vi "AUTOFLIM_Fine_Alignment.vi"(0 "System no.":i32, 5 "Scan Termination":T1(ring)=enum."Center of scan", 11 "error in":errorcluster) -> (4 "Mesh out":dbl, 6 "Numeric 2":dbl, 8 "Numeric":dbl, 10 "Alignment Array Out":dbl[][](array[numeric]), 15 "error out":errorcluster)   [LabVIEW 2023]
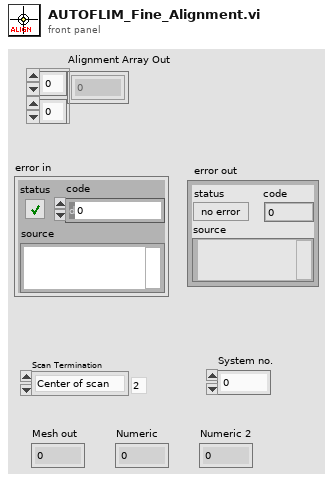
[diagram p1: front panel]
types:
  T1 = enum16{"Maximum", "End Position", "Center of scan"}
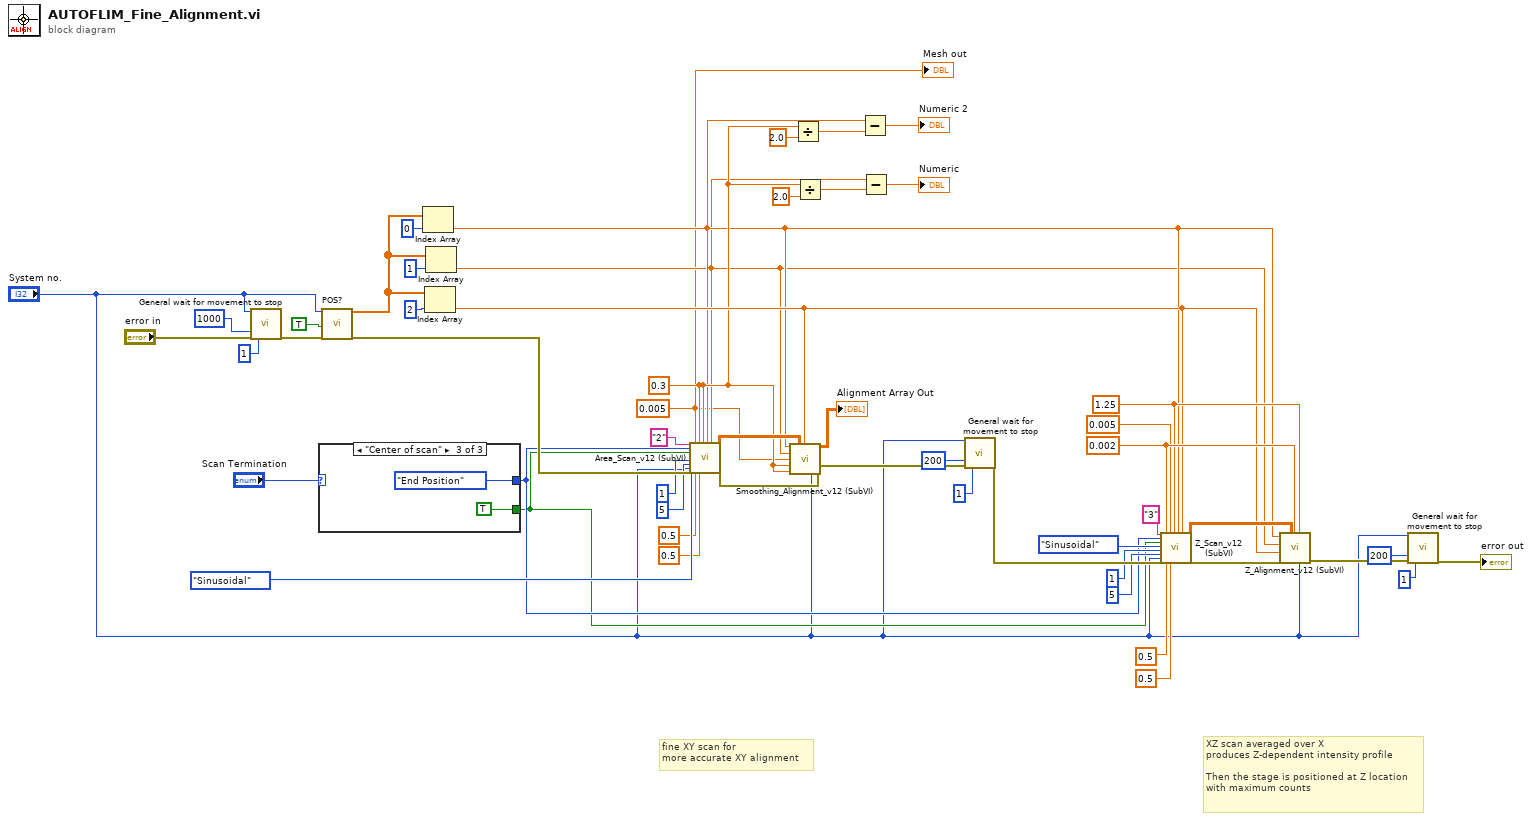
[diagram p0: block diagram]
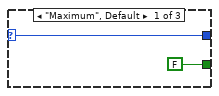
[diagram p2: hidden frame]
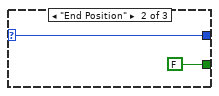
[diagram p3: hidden frame]
diagram:
  w23 = 0.002 ("Z Mesh")
  w21 = 1.25 ("Z range")
  w10 = 0.3
  w1 = 0.005
  # "fine XY scan for\nmore accurate XY alignment"
  # "XZ scan averaged over X\nproduces Z-dependent intensity profile\n\nThen the stage is positioned at Z location\nwith maximum counts"
  n1 = call "General wait for movement to stop.vi"("System no."="System no.", "Additional wait time, ms"=1000, "error in"="error in", "Polling cycle \ntime, ms"=1) -> ("error out"=w51:errorcluster)  [unwired: 4 in, 11 out]
  n2 = case shown="\"Center of scan\"" "Scan Termination" {
    selector: "Scan Termination" -> [w55 w57 _]
    tunnel: [w55 w57 T1."End Position" ("Scan Termination")] -> w25
    tunnel: [FALSE FALSE TRUE] -> w24
    frame "Maximum", Default {
    }
    frame "End Position" {
    }
    frame "Center of scan" {
    }
  }
  n3 = call "POS?.vi"("System no."="System no.", "All axes?"=TRUE, "error in"=w51) -> ("Position"=w39:dbl[], "error out"=w37:errorcluster)  [unwired: 2 in, 13 out]
  n4 = Index Array(array=w39, index=0) -> (element=w7:dbl)
  n5 = Index Array(array=w39, index=2) -> (element=w18:dbl)
  n6 = Index Array(array=w39, index=1) -> (element=w3:dbl)
  n7 = call "Area_Scan_v12 (SubVI).vi"("Step Axis"="2", "Scan Termination"=w25, "Center of Scan"=w24, "Scan Type"=enum16{"Sinusoidal", "Spiral"}."Sinusoidal", "Analog Input"=1, "Table rate"=5, "System no."="System no.", "error in (no error)"=w37, "Mesh in"=w1, "X-frequency"=0.5, "X Scan Range"=w10, "Y-velocity"=0.5, "Y Scan Range"=w10, "X Scan Center"=w7, "Y Scan Center"=w3) -> ("Intensity Graph"=w46:dbl[][], "error out"=w49:errorcluster)  [unwired: 8 in, 3 out]
  n8 = call "Smoothing_Alignment_v12 (SubVI).vi"("X center"=w7, "Intensity Graph"=w46, "Y center"=w3, "Mesh"=w1, "X Scan Range"=w10, "Y Scan Range"=w10, "Z"=w18, "System no."="System no.", "error in (no error)"=w49) -> ("Alignment Graph"=→"Alignment Array Out":dbl[][], "error out"=w32:errorcluster)  [unwired: 5 in]
  n9 = Divide(x=w10, y=2.0) -> (x/y=w6:dbl)
  n10 = Divide(x=w10, y=2.0) -> (x/y=w4:dbl)
  n11 = Subtract(x=w7, y=w6) -> (x-y=→"Numeric 2":dbl)
  n12 = Subtract(x=w3, y=w4) -> (x-y=→"Numeric":dbl)
  n13 = call "General wait for movement to stop.vi"("System no."="System no.", "Additional wait time, ms"=200, "error in"=w32, "Polling cycle \ntime, ms"=1) -> ("error out"=w29:errorcluster)  [unwired: 4 in, 11 out]
  n14 = call "Z_Scan_v12 (SubVI).vi"("Scan Axis"="3", "Scan Termination"=w25, "Center of Scan"=w24, "Scan Type"=enum16{"Sinusoidal", "Spiral"}."Sinusoidal", "Analog Input"=1, "Table rate"=5, "System no."="System no.", "error in (no error)"=w29, "Z Mesh"=w23, "Z-frequency"=0.5, "X Scan Range"=0.005, "Z-velocity"=0.5, "Z Scan Range"=w21, "X Scan Center"=w7, "Z Scan Center"=w18) -> ("Intensity Graph"=w47:dbl[][], "error out"=w48:errorcluster)  [unwired: 8 in, 3 out]
  n15 = call "Z_Alignment_v12 (SubVI).vi"("System no."="System no.", "Z range"=w21, "Intensity Graph"=w47, "Z Mesh"=w23, "error in (no error)"=w48, "Z"=w18, "Y"=w3, "X"=w7) -> ("error out"=w17:errorcluster)  [unwired: 2 in, 1 out]
  n16 = call "General wait for movement to stop.vi"("System no."="System no.", "Additional wait time, ms"=200, "error in"=w17, "Polling cycle \ntime, ms"=1) -> ("error out"=→"error out":errorcluster)  [unwired: 4 in, 11 out]
  "Mesh out" <- w1
